vi "CallWebserviceSoap.vi"(0 "reference in":refnum<class "VdTcpIP.lvclass">, 1 "MethodName":string, 2 "Arguments":string[](array[string]), 3 "ArgumentValues":string[](array[string]), 5 "error in (no error)":errorcluster, 6 "WebServicesURL_Location(Default)":string, 7 "timeout ms (25000)":i32=25000) -> (14 "reference out":refnum<class "VdTcpIP.lvclass">, 15 "Response":string, 19 "error out":errorcluster)   [LabVIEW 2020, in "VdTcpIP.lvclass"]
uses:
  VdTcpIP.lvclass
panel:
  out "concatenated string":string
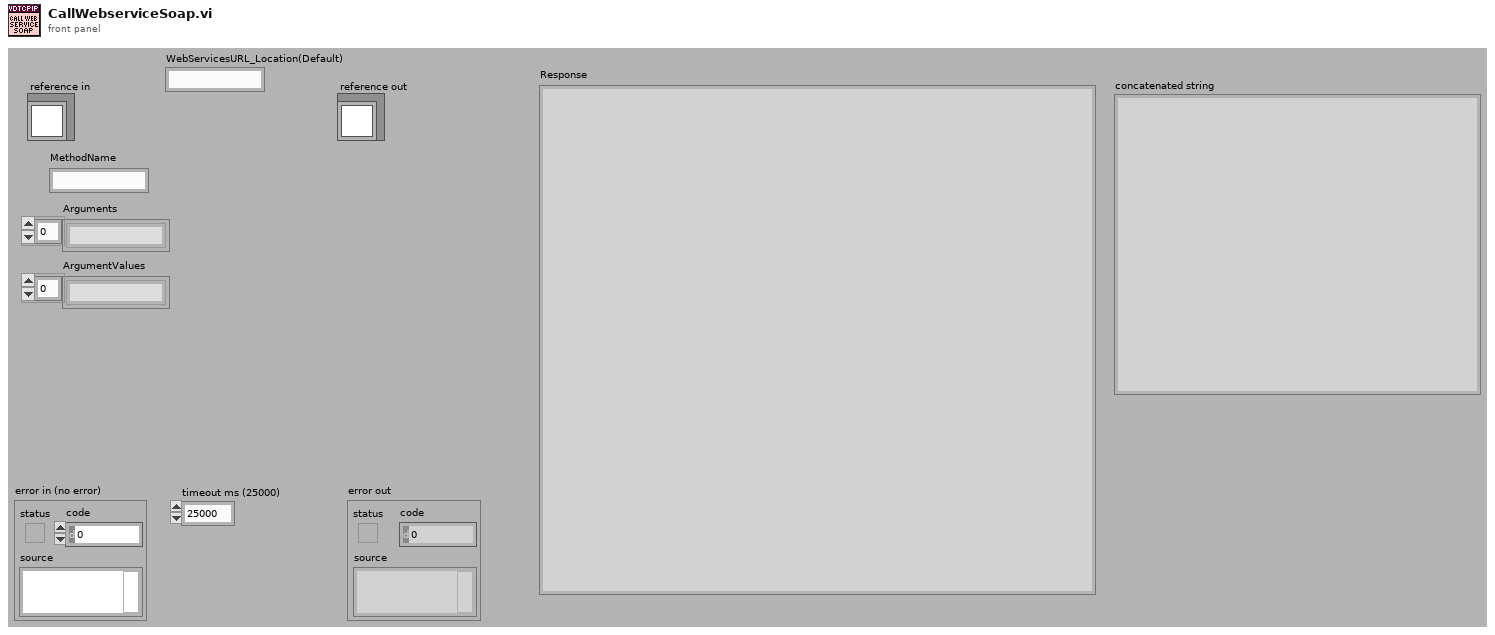
[diagram p1: front panel]
types:
  T1 = typedef "VdTcpIP.lvclass/ObjectAttributes.ctl" = cluster{"IP-Address":string, "Port":u16, "Connection":refnum<k5>, "Listener":refnum<k5>, "ListenerConnection":refnum<k5>, "Listner":bool, "ListnerProcessRunning":bool, "InConnections":refnum<k5>[], "InConnectionsIP":string[], "InConnectionAdded":refnum<notifier>, "RunVIOnNewConnection":variant, "DataToNewConnectionVI":cluster{"ControlName":string, "ControlValue":variant}[], "WebServicesURL_Location(http://...)":string, "WebServicesPostWebPage(*.asmx)":string, "Semaphore":T2, "AutoReConnectTimes":i32, "AutoReConnectInterval(ms)":i32, "ConnectionTimeout":i32}
  T2 = typedef "Semaphore RefNum" = refnum<k1>
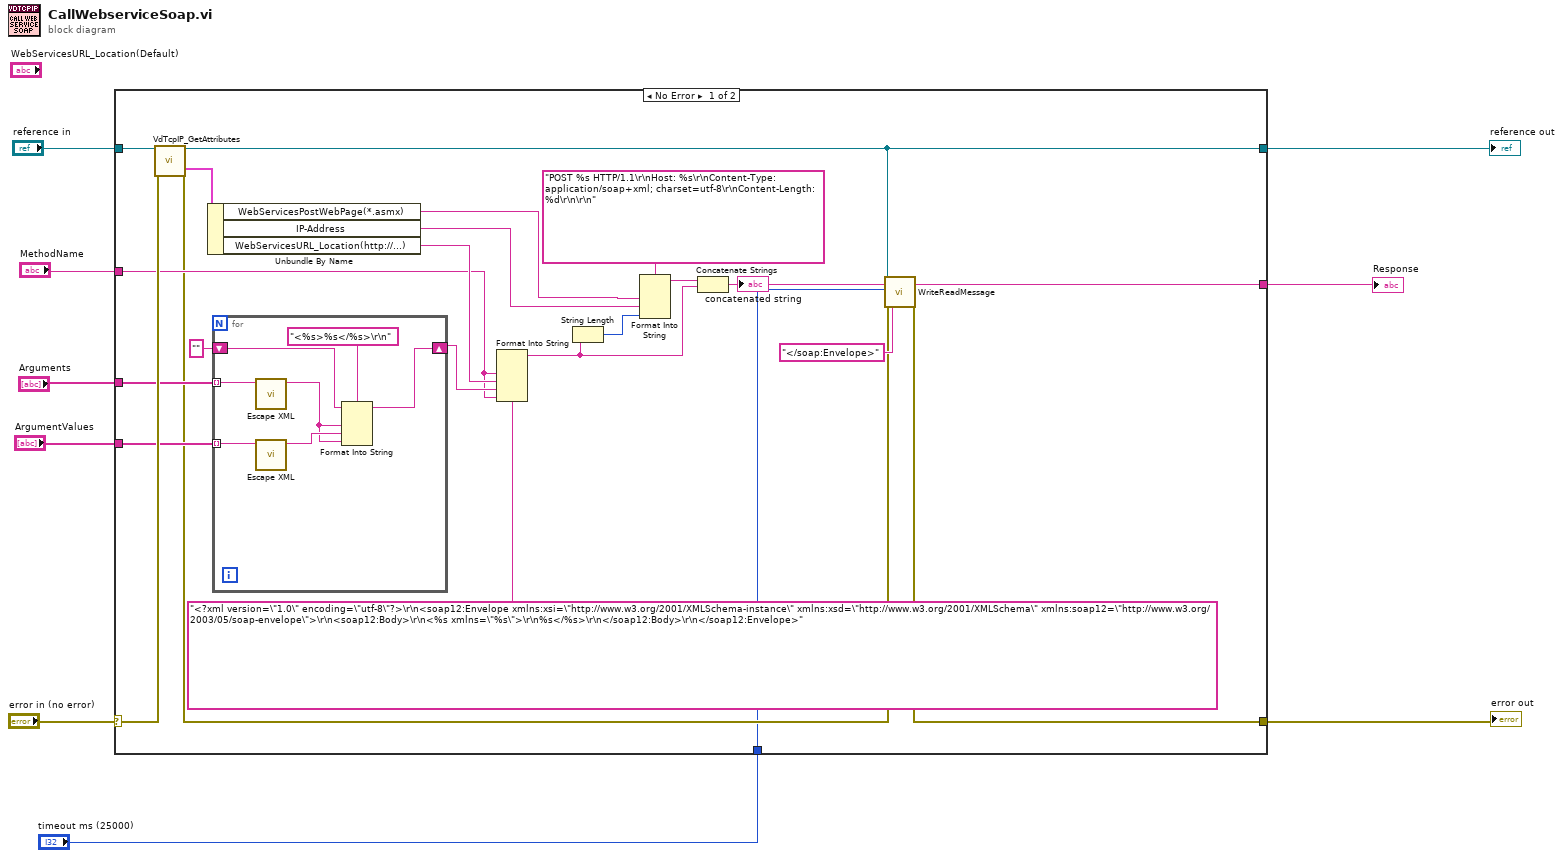
[diagram p0: block diagram]
diagram:
  n1 = case shown="No Error" "error in (no error)" {
    selector: "error in (no error)" -> [w32 w41]
    tunnel: [w16 w41] -> w8
    tunnel: [w18 w40] -> w6
    tunnel: "reference in" -> [w31 w40]
    tunnel: "Arguments" -> [w30 _]
    tunnel: "ArgumentValues" -> [w29 _]
    tunnel: "MethodName" -> [w21 _]
    tunnel: "timeout ms (25000)" -> [w15 _]
    tunnel: [w14 _] -> w1
    frame No Error {
      n2 = call "VdTcpIP_GetAttributes.vi"("reference in"=w31, "error in (no error)"=w32) -> ("reference out"=w18:refnum<class "VdTcpIP.lvclass">, "Data"=w10:T1, "error out"=w17:errorcluster)  [unwired: 1 in, 14 out]
      n3 = Unbundle By Name(w10) -> ("WebServicesPostWebPage(*.asmx)"=w12:string, "IP-Address"=w13:string, "WebServicesURL_Location(http://...)"=w23:string)
      n4 = for {
        tunnel: w30 -> [w39] mode=indexing
        tunnel: w29 -> [w38] mode=indexing
        shift-right: [w33] -> w22
        shift-left: "" -> [w34]
        n5 = call <vilib>:"Escape XML.vi"("XML String In"=w39) -> ("XML String Out"=w35:string)  [unwired: 1 in, 9 out]
        n6 = call <vilib>:"Escape XML.vi"("XML String In"=w38) -> ("XML String Out"=w36:string)  [unwired: 1 in, 9 out]
        n7 = Format Into String(format string="<%s>%s</%s>\r\n", initial string=w34, w35, w36, w35) -> (resulting string=w33:string)  [unwired: 1 in, 1 out]
      }
      n8 = Format Into String(format string="<?xml version=\"1.0\" encoding=\"utf-8\"?>\r\n<soap12:Envelope xmlns:xsi=\"http://www.w3.org/2001/XMLSchema-instance\" xmlns:xsd=\"http://www.w3.org/2001/XMLSchema\" xmlns:soap12=\"http://www.w3.org/2003/05/soap-envelope\">\r\n<soap12:Body>\r\n<%s xmlns=\"%s\">\r\n%s</%s>\r\n</soap12:Body>\r\n</soap12:Envelope>", w21, w23, w22, w21) -> (resulting string=w20:string)  [unwired: 2 in, 1 out]
      n9 = String Length(string=w20) -> (length=w26:i32)
      n10 = Format Into String(format string="POST %s HTTP/1.1\r\nHost: %s\r\nContent-Type: application/soap+xml; charset=utf-8\r\nContent-Length: %d\r\n\r\n", w12, w13, w26) -> (resulting string=w25:string)  [unwired: 2 in, 1 out]
      n11 = Concatenate Strings(w25, w20) -> (w11:string)
      "concatenated string" <- w11
      n12 = call "WriteReadMessage.vi"("reference"=w18, "MessageToWrite"=w11, "timeout ms (25000)"=w15, "error in (no error)"=w17, "ReadUntilDataReceived(Ignored if not wired)"="</soap:Envelope>") -> ("ReturnedMessage"=w14:string, "error out"=w16:errorcluster)  [unwired: 2 in, 11 out]
    }
    frame Error {
    }
  }
  "error out" <- w8
  "reference out" <- w6
  "Response" <- w1
